vi "getOffsetToUTC.vi"(11 "Epoch":refnum<class "Epoch.UTC.lvclass">) -> (2 "Offset to UTC":i64)   [LabVIEW 2013, in "Epoch.UTC.lvclass"]
uses:
  Epoch.UTC.lvclass
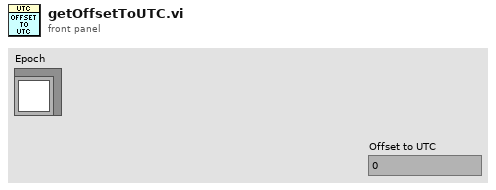
[diagram p1: front panel]
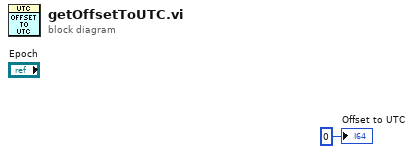
[diagram p0: block diagram]
diagram:
  "Offset to UTC" <- i64 0 ("Offset to UTC")
